vi "Map Axis.vi"(8 "error in (no error)":errorcluster, 10 "Array":refnum<class "iMotion Controller.lvclass">[](array[class]), 11 "MAS in":refnum<class "MAS.lvclass">) -> (0 "error out":errorcluster, 3 "MAS out":refnum<class "MAS.lvclass">)   [LabVIEW 2022 SP3, in "MAS.lvclass"]
uses:
  MAS.lvclass
  iMotion Controller/iMotion Controller.lvclass
  MAS.lvclass/MAS.ctl
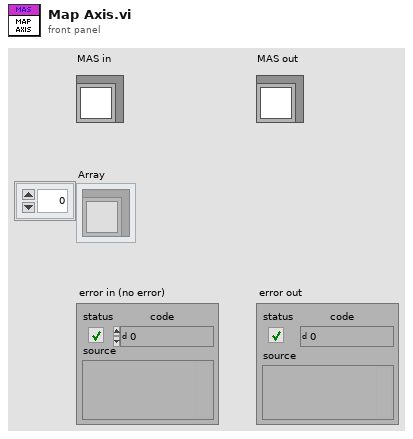
[diagram p1: front panel]
types:
  T1 = map{string, refnum<class "iMotion Controller.lvclass">}
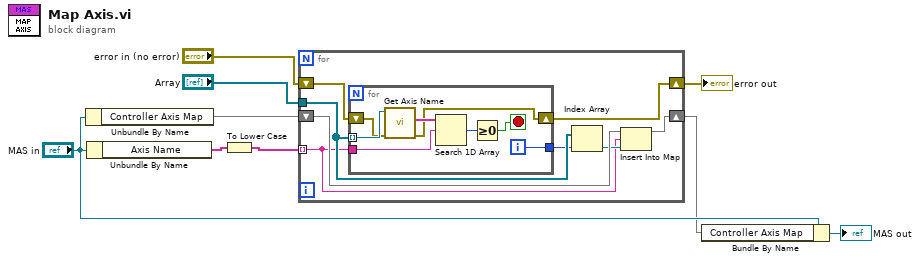
[diagram p0: block diagram]
diagram:
  n1 = Unbundle By Name("MAS in") -> ("Controller Axis Map"=w9:T1)
  n2 = Unbundle By Name("MAS in") -> ("Axis Name"=w2:string[])
  n3 = To Lower Case(string=w2) -> (all lower case string=w1:string[])
  n4 = for {
    tunnel: "Array" -> [w15]
    tunnel: w1 -> [w12] mode=indexing
    shift-right: [w16] -> w7
    shift-left: w9 -> [w17]
    shift-right: [w10] -> w3
    shift-left: "error in (no error)" -> [w11]
    n5 = for {
      tunnel: w12 -> [w24]
      tunnel: w15 -> [w23] mode=indexing
      tunnel: [w22] -> w14
      shift-right: [w18] -> w10
      shift-left: w11 -> [w19]
      i -> [w22]
      stop <- w20 stop-if-true
      n6 = call-dynamic "Get Axis Name.vi"("error in (no error)"=w19, "iMotion Controller in"=w23) -> ("error out"=w18:errorcluster, "Axis Name"=w25:string[])  [unwired: 7 in, 1 out]
      n7 = Search 1D Array(1D array=w25, element=w24) -> (index of element=w21:i32)  [unwired: 1 in]
      n8 = Greater Or Equal To 0?(x=w21) -> (x >= 0?=w20:bool)
    }
    n9 = Index Array(array=w15, index=w14) -> (element=w13:refnum<class "iMotion Controller.lvclass">)
    n10 = Insert Into Map(map in=w17, key=w12, value=w13) -> (map out=w16:T1)  [unwired: 2 out]
  }
  "error out" <- w3
  n11 = Bundle By Name(cluster="MAS in", "Controller Axis Map"=w7) -> (→"MAS out":refnum<class "MAS.lvclass">)
